vi "Connect.vi"(6 "Format":T1, 8 "error in (no error)":errorcluster, 10 "Stream:Connection":refnum<class "Connection.lvclass">, 11 "Manager in":refnum<class "Manager.lvclass">) -> (0 "error out":errorcluster, 2 "Endpoint":refnum<class "Endpoint.lvclass">, 3 "Manager out":refnum<class "Manager.lvclass">)   [LabVIEW 2020, in "Stream-Simple-Msg.lvlib" / "Manager.lvclass"]
uses:
  Manager.lvclass
  <vilib>/IlluminatedG/lv-stream/Connection/Connection.lvclass
  C:/Program Files (x86)/National Instruments/LabVIEW 2020/vi.lib/IlluminatedG/lv-stream/Endpoint/Endpoint.lvclass
  Endpoint/Endpoint.lvclass
  Format.ctl
  Mapped Endpoint.ctl
  Manager.lvclass/Manager.ctl
  <vilib>/IlluminatedG/lv-stream/Endpoint/Endpoint.lvclass
  <vilib>/IlluminatedG/lv-stream/URI/URI.lvclass
  Stream-Simple-Msg.lvlib
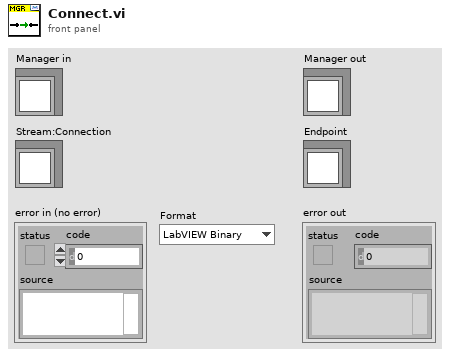
[diagram p1: front panel]
types:
  T1 = typedef "Stream-Simple-Msg.lvlib/Format.ctl" = enum16{"LabVIEW Binary", "JSON"}
  T2 = typedef "Stream-Simple-Msg.lvlib/Manager.lvclass/Mapped Endpoint.ctl" = cluster{"Msg Endpoint":refnum<class "Endpoint.lvclass">, "Format":T1}
  T3 = typedef "Stream-Simple-Msg.lvlib/Manager.lvclass/Ref Data.ctl" = cluster{"Message Callbacks":map{string, T4[]}, "Endpoints":map{string, T2}, "Stream Endpoints":refnum<class "Endpoint.lvclass">[], "State Callbacks":T5[], "Stream Formats":T1[]}
  T4 = typedef "Stream-Simple-Msg.lvlib/Manager.lvclass/Callback.ctl" = cluster{"VI":refnum<vi>, "Owner":refnum<class>}
  T5 = typedef "Stream-Simple-Msg.lvlib/Manager.lvclass/State Callback.ctl" = cluster{"Owner":refnum<class>, "VI":refnum<vi>, "Context":variant}
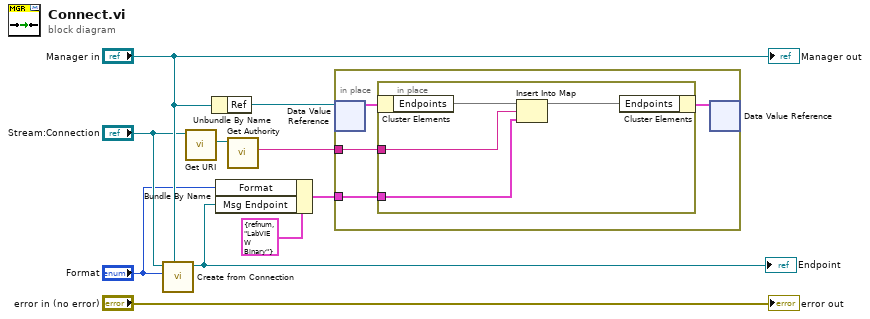
[diagram p0: block diagram]
diagram:
  n1 = call "Create from Connection.vi"("Manager"="Manager in", "Format"="Format", "Stream:Connection"="Stream:Connection") -> ("Endpoint out"=w3:refnum<class "Endpoint.lvclass">)  [unwired: 7 in, 1 out]
  "Endpoint" <- w3
  n2 = call <vilib>:"Get URI.vi"("Endpoint in"="Stream:Connection") -> ("URI"=w6:refnum<class "URI.lvclass">)  [unwired: 8 in, 2 out]
  n3 = Unbundle By Name("Manager in") -> ("Ref"=w8:refnum<data-value>)
  n4 = Bundle By Name(cluster=T2 {"Msg Endpoint"=refnum, "Format"=enum."LabVIEW Binary"} ("Mapped Endpoint"), "Format"="Format", "Msg Endpoint"=w3) -> (w1:T2)
  n5 = call <vilib>:"Get Authority.vi"("URI in"=w6) -> ("Authority"=w5:string)  [unwired: 8 in, 2 out]
  n6 = in-place {
    in-place-border: w5 -> [w13]
    in-place-border: w1 -> [w11]
    n7 = in-place-dvr #1(w8) -> (w14:T3)  [unwired: 1 out]
    n8 = in-place {
      in-place-border: w13 -> [w17]
      in-place-border: w11 -> [w15]
      n9 = in-place-cluster #2(w14) -> ("Endpoints"=w18:map{string, T2})
      n10 = Insert Into Map(map in=w18, key=w17, value=w15) -> (map out=w16:map{string, T2})  [unwired: 2 out]
      n11 = in-place-cluster #2("Endpoints"=w16) -> (w12:T3)
    }
    n12 = in-place-dvr #1(w12) -> ()  [unwired: 2 out]
  }
  "error out" <- "error in (no error)"
  "Manager out" <- "Manager in"
